vi "mppt_keithley-2450_python.vi"(0 "start voltage (V)":string, 1 "file name":string, 2 "folder path":string, 5 "nplc":string, 7 "settling delay (s)":string, 9 "total tracking time (s)":string, 11 "error in (no error)":errorcluster, 12 "illumination intensity (suns equiv.)":string, 13 "area (cm^2)":string) -> (15 "error out":errorcluster)   [LabVIEW 2016]
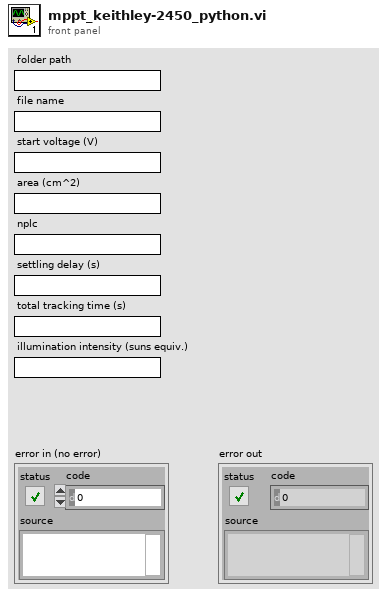
[diagram p1: front panel]
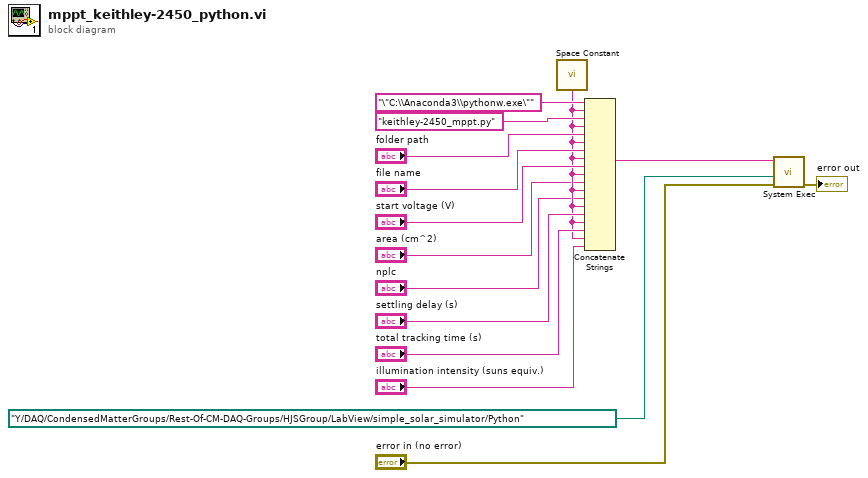
[diagram p0: block diagram]
diagram:
  n1 = call <vilib>:"Space Constant.vi"() -> ("String"=w3:string)
  n2 = Concatenate Strings("\"C:\\Anaconda3\\pythonw.exe\"" ("standard input"), w3, "keithley-2450_mppt.py" ("standard input"), w3, "folder path", w3, "file name", w3, "start voltage (V)", w3, "area (cm^2)", w3, "nplc", w3, "settling delay (s)", w3, "total tracking time (s)", w3, "illumination intensity (suns equiv.)") -> (w13:string)
  n3 = call <vilib>:"System Exec.vi"("error in (no error)"="error in (no error)", "working directory"=path "Y:/DAQ/CondensedMatterGroups/Rest-Of-CM-DAQ-Groups/HJSGroup/LabView/simple_solar_simulator/Python", "command line"=w13) -> ("error out"=→"error out":errorcluster)  [unwired: 5 in, 3 out]
